vi "StartOrEndAcquisition.vi"(0 "Start/Stop":bool, 1 "Piezo Mode":string="Live", 5 "Ready to End Acquire Rendezvous":T1, 7 "Ready To Acquire Rendezvous":T1, 9 "Acquire Chnage NOtifier":refnum<notifier>, 11 "error in":errorcluster, 12 "Laser Mode":string="Green Confocal") -> (15 "error out 2":errorcluster)   [LabVIEW 2015]
uses:
  <userlib>/atmcd64d.llb/AcquisitionMode_mode typedef.ctl
  NIDAQControls/NIDAQGlobals.vi
  AcquisitionGlobals.vi
  NIDAQControls/StateGlobals.vi
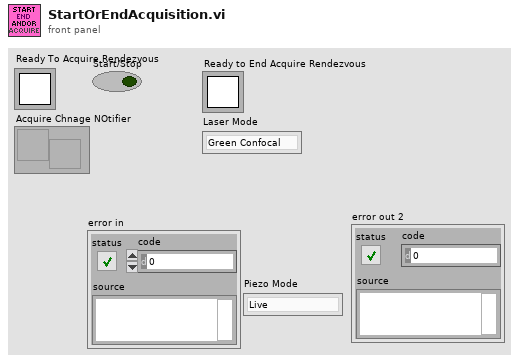
[diagram p1: front panel]
types:
  T1 = typedef "Rendezvous RefNum" = refnum<k1>
  T2 = typedef "AcquisitionMode_mode typedef.ctl" = enum16{"Reserved (0)", "Single Scan", "Accumulate", "Kinetics", "Fast Kinetics", "Run Till Abort", "Reserved (6)", "Reserved (7)", "Reserved (8)", "Time Delayed Integration"}
  T3 = cluster{"notification":bool, "Laser Mode":string, "Piezo Mode":string, "Piezo Mode":string}
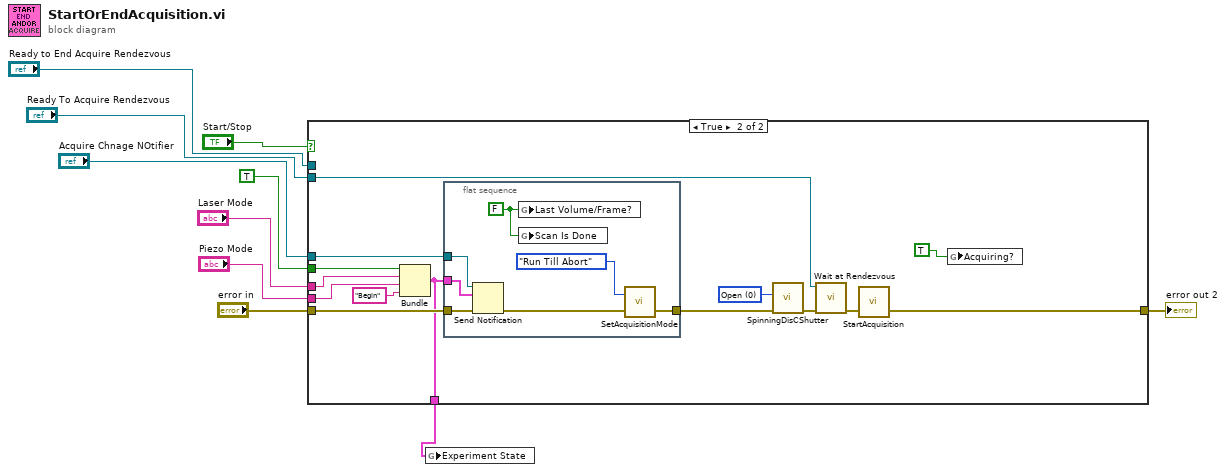
[diagram p0: block diagram]
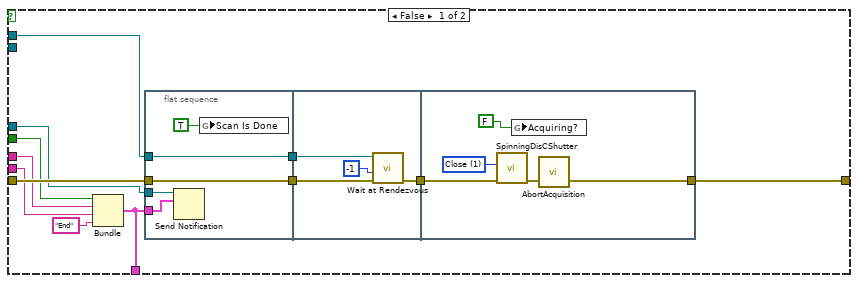
[diagram p2: hidden frame]
diagram:
  n1 = case shown="True" "Start/Stop" {
    tunnel: "error in" -> [w22 w50]
    tunnel: [w21 w47] -> w7
    tunnel: "Ready to End Acquire Rendezvous" -> [w19 _]
    tunnel: "Ready To Acquire Rendezvous" -> [_ w44]
    tunnel: "Acquire Chnage NOtifier" -> [w14 w43]
    tunnel: TRUE ("notification") -> [w16 w37]
    tunnel: "Laser Mode" -> [w17 w42]
    tunnel: "Piezo Mode" -> [w15 w41]
    tunnel: [w13 w39] -> w1
    frame False {
      n2 = Bundle("notification"=w16, "Laser Mode"=w17, "Piezo Mode"=w15, "Piezo Mode"="End") -> (w13:T3)  [unwired: 1 in]
      n3 = flat-sequence {
        tunnel: w22 -> [w26]
        tunnel: [w26] -> w12
        tunnel: w19 -> [w27]
        tunnel: [w27] -> w11
        tunnel: w14 -> [w25]
        tunnel: w13 -> [w24]
        tunnel: w12 -> [w28]
        tunnel: [w31] -> w20
        tunnel: w11 -> [w29]
        tunnel: w20 -> [w35]
        tunnel: [w36] -> w21
        frame #0 {
          n4 = Send Notification(notification=w24, notifier=w25) -> ()  [unwired: 1 in, 2 out]
          n5 = global write "NIDAQGlobals.vi" "Scan Is Done"(TRUE ("Last Volume/Frame?")) -> ()
        }
        frame #1 {
          n6 = call <vilib>:"Wait at Rendezvous.vi"("error in (no error)"=w28, "ms timeout (-1)"=-1 ("timeout in ms (-1)"), "rendezvous"=w29) -> ("error out"=w31:errorcluster)  [unwired: 2 in, 2 out]
        }
        frame #2 {
          w33 = u16 1 items=["Open", "Close"] ("Ring")
          n7 = call "SpinningDisCShutter.vi"("error in (no error)"=w35, "Ring"=w33) -> ("error out"=w34:errorcluster)  [unwired: 9 in]
          n8 = global write "AcquisitionGlobals.vi" "Acquiring?"(FALSE) -> ()
          n9 = call <userlib>:"AbortAcquisition.vi"("error in (no error)"=w34) -> ("error out"=w36:errorcluster)  [unwired: 1 in, 1 out]
        }
      }
    }
    frame True {
      w49 = u16 0 items=["Open", "Close"] ("Ring")
      n10 = Bundle("notification"=w37, "Laser Mode"=w42, "Piezo Mode"=w41, "Piezo Mode"="Begin") -> (w39:T3)  [unwired: 1 in]
      n11 = flat-sequence {
        tunnel: w50 -> [w56]
        tunnel: [w54] -> w48
        tunnel: w43 -> [w52]
        tunnel: w39 -> [w51]
        frame #0 {
          w53 = FALSE ("Last Volume/Frame?")
          n12 = Send Notification(notification=w51, notifier=w52, error in (no error)=w56) -> (error out=w55:errorcluster)  [unwired: 1 out]
          n13 = global write "NIDAQGlobals.vi" "Last Volume/Frame?"(w53) -> ()
          n14 = global write "NIDAQGlobals.vi" "Scan Is Done"(w53) -> ()
          n15 = call <userlib>:"SetAcquisitionMode.vi"("error in (no error)"=w55, "mode"=AcquisitionMode_mode_typedef."Run Till Abort") -> ("error out"=w54:errorcluster)  [unwired: 1 out]
        }
      }
      n16 = call "SpinningDisCShutter.vi"("error in (no error)"=w48, "Ring"=w49) -> ("error out"=w46:errorcluster)  [unwired: 9 in]
      n17 = call <vilib>:"Wait at Rendezvous.vi"("error in (no error)"=w46, "rendezvous"=w44) -> ("error out"=w45:errorcluster)  [unwired: 3 in, 2 out]
      n18 = call <userlib>:"StartAcquisition.vi"("error in (no error)"=w45) -> ("error out"=w47:errorcluster)  [unwired: 1 in, 1 out]
      n19 = global write "AcquisitionGlobals.vi" "Acquiring?"(TRUE) -> ()
    }
  }
  "error out 2" <- w7
  n20 = global write "StateGlobals.vi" "Experiment State"(w1) -> ()
